vi "Create DVR.vi"(8 "Error In":errorcluster) -> (0 "Error Out":errorcluster, 2 "DVR Ref":T1[](array[typedef]), 3 "Class Names":string[](array[string]))   [LabVIEW 2023, in "Message Data.lvclass"]
uses:
  Message Data.lvclass
  Controls/Class DVR Ref.ctl
  Message Data.lvclass/Message Data.ctl
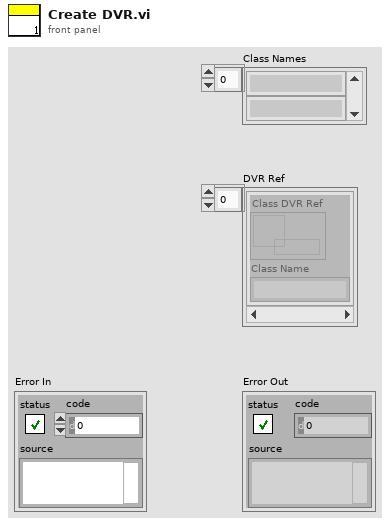
[diagram p1: front panel]
types:
  T1 = typedef "Class DVR Ref.ctl" = cluster{"Class DVR Ref":refnum<data-value>, "Class Name":string}
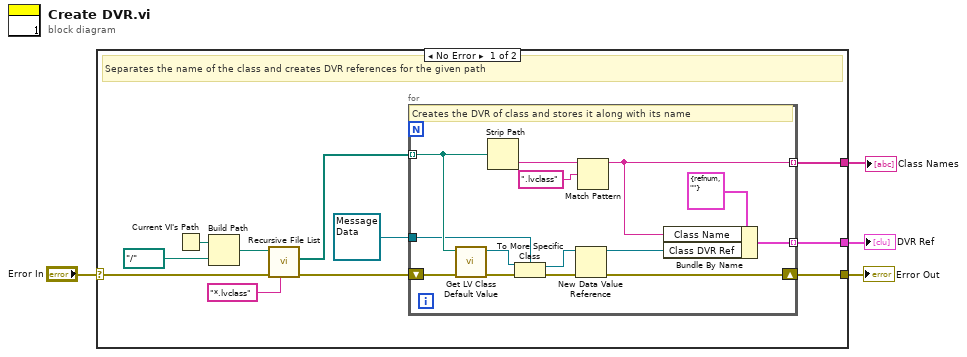
[diagram p0: block diagram]
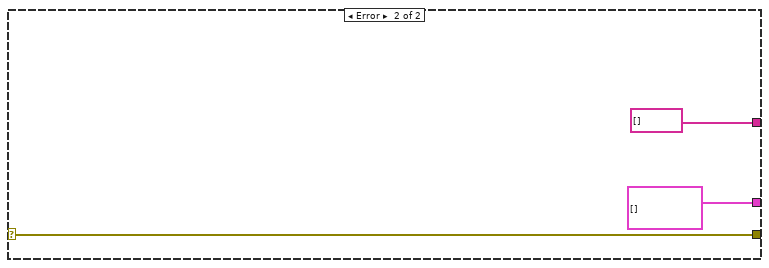
[diagram p2: hidden frame]
diagram:
  n1 = case shown="No Error" "Error In" {
    selector: "Error In" -> [w7 w32]
    tunnel: [w14 w32] -> w3
    tunnel: [w13 string[] []] -> w2
    tunnel: [w12 T1[] []] -> w1
    frame No Error {
      # "Separates the name of the class and creates DVR references for the given path"
      n2 = Current VI's Path() -> (path=w10:path)
      n3 = Build Path(base path=w10, name or relative path=path "../..") -> (appended path=w9:path)
      n4 = call <vilib>:"Recursive File List.vi"("pattern"="*.lvclass", "error in (no error)"=w7, "Folder Path"=w9) -> ("error out"=w6:errorcluster, "All Files in Dir"=w5:path[])  [unwired: 4 in, 3 out]
      n5 = for {
        tunnel: w5 -> [w26] mode=indexing
        tunnel: [w16] -> w13 mode=indexing
        shift-right: [w22] -> w14
        shift-left: w6 -> [w28]
        tunnel: refnum<class "Message Data.lvclass"> refnum ("Arithemetic Operation in") -> [w25]
        tunnel: [w17] -> w12 mode=indexing
        # "Creates the DVR of class and stores it along with its name"
        n6 = call <vilib>:"Get LV Class Default Value.vi"("error in (no error)"=w28, "class path"=w26) -> ("error out"=w27:errorcluster, "object"=w24:refnum<class>)  [unwired: 8 in]
        n7 = Strip Path(path=w26) -> (name=w20:string)  [unwired: 1 out]
        n8 = To More Specific Class(target class=w25, reference=w24, error in=w27) -> (specific class reference=w21:refnum<class "Message Data.lvclass">, error out=w23:errorcluster)
        n9 = New Data Value Reference(data value=w21, error in=w23) -> (data value reference=w19:refnum<data-value>, error out=w22:errorcluster)
        n10 = Match Pattern(string=w20, regular expression=".lvclass") -> (before substring=w16:string)  [unwired: 1 in, 3 out]
        n11 = Bundle By Name(cluster=T1 {"Class DVR Ref"=refnum, "Class Name"=""}, "Class Name"=w16, "Class DVR Ref"=w19) -> (w17:T1)
      }
    }
    frame Error {
    }
  }
  "Error Out" <- w3
  "DVR Ref" <- w1
  "Class Names" <- w2
